vi "Table, Set Column Value, String.vi"(6 "column (0)":i32, 8 "error in":errorcluster, 10 "Value":string[](array[string]), 11 "Tbl Refnum":refnum<vi>) -> (0 "error out":errorcluster, 3 "Tbl Refnum out":refnum<vi>, 4 "column+1":i32)   [LabVIEW 2010]
doc: "Converts one row from a Test Criteria Table to a TestStand Result cluster."
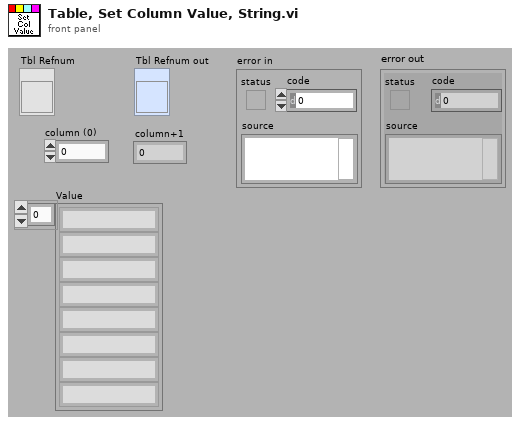
[diagram p1: front panel]
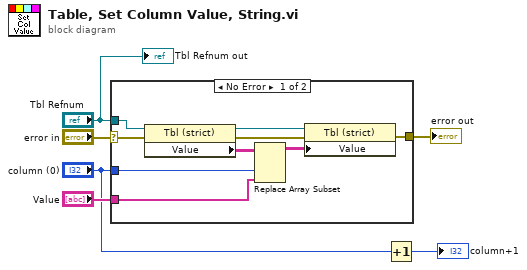
[diagram p0: block diagram]
diagram:
  n1 = case shown="No Error" "error in" {
    selector: "error in" -> [w14 w16]
    tunnel: "Tbl Refnum" -> [w15 _]
    tunnel: [w13 w16] -> w6
    tunnel: "column (0)" -> [w9 _]
    tunnel: "Value" -> [w8 _]
    frame No Error {
      n2 = property class="Tbl (strict)"(reference=w15, error in=w14) -> (reference out=w7:refnum<vi>, error out=w12:errorcluster, "Value"=w10:string[][])
      n3 = Replace Array Subset(array=w10, new element=w8, index (col)=w9) -> (w11:string[][])  [unwired: 1 in]
      n4 = property class="Tbl (strict)"(reference=w7, error in=w12, "Value"=w11) -> (error out=w13:errorcluster)  [unwired: 1 out]
    }
    frame Error {
    }
  }
  "error out" <- w6
  n5 = Increment(x="column (0)") -> (x+1=→"column+1":i32)
  "Tbl Refnum out" <- "Tbl Refnum"
